vi "Set Output.vi"(8 "error in (no error)":errorcluster, 10 "Output value":refnum<class "Mag Lab Result.lvclass">, 11 "Mag Lab Temperature Controller in":refnum<class "Mag Lab Temperature Controller.lvclass">) -> (0 "error out":errorcluster, 2 "Actual output value":refnum<class "Mag Lab Result.lvclass">, 3 "Mag Lab Temperature Controller out":refnum<class "Mag Lab Temperature Controller.lvclass">)   [LabVIEW 2015, in "Mag Lab Temperature Controller.lvclass"]
uses:
  Mag Lab Temperature Controller.lvclass
  Mag Lab Result/Mag Lab Result.lvclass
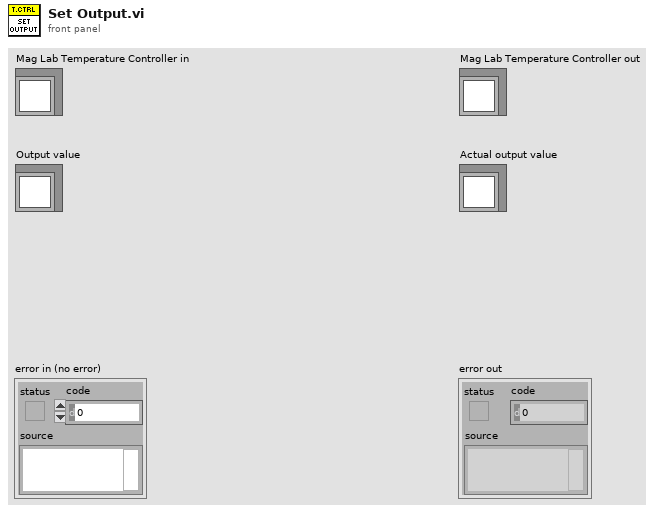
[diagram p1: front panel]
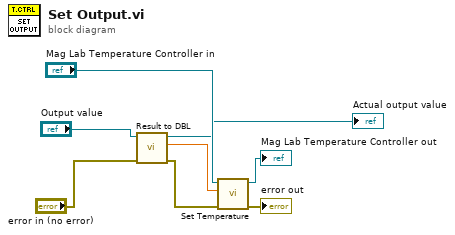
[diagram p0: block diagram]
diagram:
  n1 = call "Result to DBL.vi"("error in (no error)"="error in (no error)", "Mag Lab Result"="Output value") -> ("error out"=w4:errorcluster, "Value"=w3:dbl, "Mag Lab Result out"=→"Actual output value":refnum<class "Mag Lab Result.lvclass">)  [unwired: 7 in]
  n2 = call-dynamic "Set Temperature.vi"("error in (no error)"=w4, "Set temperature"=w3, "Mag Lab Temperature Controller in"="Mag Lab Temperature Controller in") -> ("error out"=→"error out":errorcluster, "Mag Lab Temperature Controller out"=→"Mag Lab Temperature Controller out":refnum<class "Mag Lab Temperature Controller.lvclass">)  [unwired: 7 in]
